vi "Error Not Implemented.vi"(8 "error in (no error)":errorcluster) -> (0 "error out":errorcluster)   [LabVIEW 2020, in "Stream.lvlib"]
uses:
  Stream.lvlib
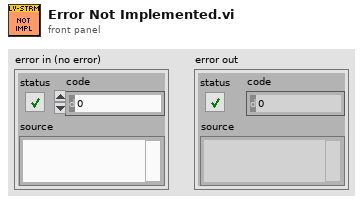
[diagram p1: front panel]
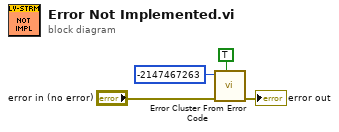
[diagram p0: block diagram]
diagram:
  n1 = call <vilib>:"Error Cluster From Error Code.vi"("show call chain? (False)"=TRUE, "error in (no error)"="error in (no error)", "error code (0)"=-2147467263) -> ("error out"=→"error out":errorcluster)  [unwired: 6 in]
